vi "Block Name.vi"(8 "error in (no error)":errorcluster, 11 "Block in":refnum<class "Block.lvclass">) -> (0 "error out":errorcluster, 2 "Name":string, 3 "Block out":refnum<class "Block.lvclass">)   [LabVIEW 2020, in "Parallel Block.lvlib" / "Block.lvclass"]
uses:
  Block.lvclass
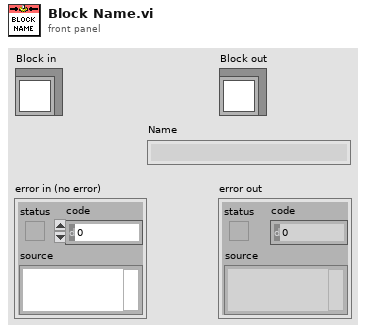
[diagram p1: front panel]
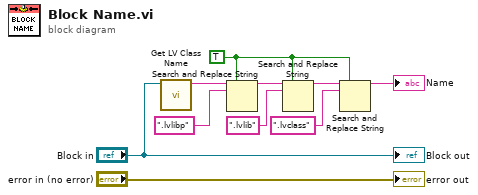
[diagram p0: block diagram]
diagram:
  w4 = TRUE ("replace all? (F)")
  n1 = call <vilib>:"Get LV Class Name.vi"("object"="Block in") -> ("class name"=w8:string)  [unwired: 9 in, 1 out]
  n2 = Search and Replace String(replace all?=w4, input string=w8, search string=".lvlibp") -> (result string=w6:string)  [unwired: 5 in, 3 out]
  n3 = Search and Replace String(replace all?=w4, input string=w6, search string=".lvlib") -> (result string=w3:string)  [unwired: 5 in, 3 out]
  n4 = Search and Replace String(replace all?=w4, input string=w3, search string=".lvclass") -> (result string=→"Name":string)  [unwired: 5 in, 3 out]
  "error out" <- "error in (no error)"
  "Block out" <- "Block in"
